vi "linkdln day 1 vi.vi"() -> ()   [LabVIEW 2022 SP3]
panel:
  in  "stop":bool
  out "Numeric Indicator":dbl
  in  "Numeric Control 2":dbl
  in  "Numeric Control":dbl
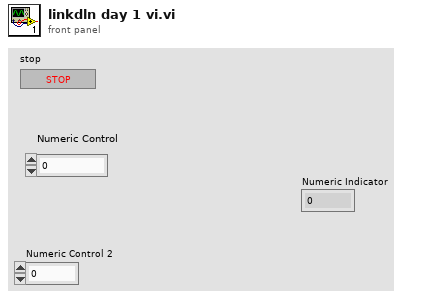
[diagram p1: front panel]
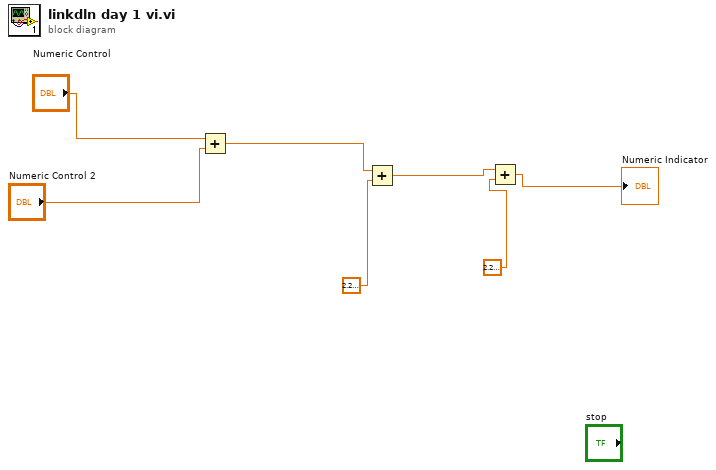
[diagram p0: block diagram]
diagram:
  n1 = Add(x="Numeric Control", y="Numeric Control 2") -> (x+y=w5:dbl)
  n2 = Add(x=w5, y=2.220446049250313e-16) -> (x+y=w3:dbl)
  n3 = Add(x=w3, y=2.220446049250313e-16) -> (x+y=→"Numeric Indicator":dbl)
